vi "get channels.vi"(11 "alarms module configuration in":refnum<class "alarms module configuration.lvclass">) -> (2 "channels":refnum<class "TBM channel.lvclass">[](array[class]), 3 "alarms module configuration out":refnum<class "alarms module configuration.lvclass">)   [LabVIEW 2013, in "alarms module configuration.lvclass"]
uses:
  alarms module configuration.lvclass
  <vilib>/NI/Tag Bus Module Framework/channel/TBM channel.lvclass
  alarms module configuration.lvclass/alarms module configuration.ctl
  <vilib>/NI/Tag Bus/tag/tag descriptor.lvclass/tag descriptor.ctl
  <vilib>/NI/Tag Bus/tag/tag descriptor.lvclass
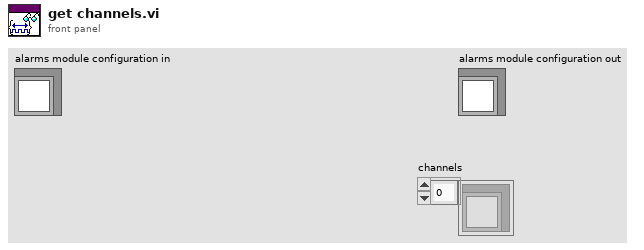
[diagram p1: front panel]
types:
  T1 = typedef "alarms module configuration.lvclass/alarm configuration.ctl" = cluster{"alarm name":string, "comparisons":T2[], "unlatch":refnum<class "TBM channel.lvclass">, "output":refnum<class "TBM channel.lvclass">, "boolean op":T4}
  T2 = typedef "alarms module configuration.lvclass/alarm comparison.ctl" = cluster{"input channel":refnum<class "TBM channel.lvclass">, "limit":dbl, "comparison":T3}
  T3 = typedef "alarms module configuration.lvclass/compare type.ctl" = enum16{">", "<", ">=", "<=", "="}
  T4 = typedef "alarms module configuration.lvclass/boolean operation.ctl" = enum16{"AND", "OR"}
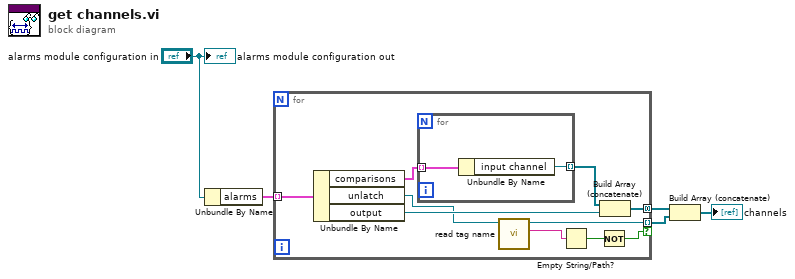
[diagram p0: block diagram]
diagram:
  n1 = Unbundle By Name("alarms module configuration in") -> ("alarms"=w4:T1[])
  n2 = for {
    tunnel: w4 -> [w13] mode=indexing
    tunnel: [w14] -> w3 mode=concatenating
    tunnel: [w9] -> w1 mode=indexing if=w6
    n3 = Unbundle By Name(w13) -> ("comparisons"=w11:T2[], "unlatch"=w10:refnum<class "TBM channel.lvclass">, "output"=w12:refnum<class "TBM channel.lvclass">)
    n4 = for {
      tunnel: [w17] -> w15 mode=indexing
      tunnel: w11 -> [w16] mode=indexing
      n5 = Unbundle By Name(w16) -> ("input channel"=w17:refnum<class "TBM channel.lvclass">)
    }
    n6 = call <vilib>:"read tag name.vi"("system tag in"=w10) -> ("name"=w8:string, "system tag out"=w9:refnum<class "TBM channel.lvclass">)  [unwired: 8 in, 1 out]
    n7 = Empty String/Path?(string/path=w8) -> (empty?=w7:bool)
    n8 = Not(x=w7) -> (.not. x?=w6:bool)
    n9 = Build Array (concatenate)(w15, w12) -> (w14:refnum<class "TBM channel.lvclass">[])
  }
  n10 = Build Array (concatenate)(w3, w1) -> (→"channels":refnum<class "TBM channel.lvclass">[])
  "alarms module configuration out" <- "alarms module configuration in"
